vi "HW_QX_Parse Channel Parameters.vi"(8 "error in":errorcluster, 10 "sysModCFG[]":T1[](array[typedef])) -> (0 "error out":errorcluster)   [LabVIEW 2016]
uses:
  Ctrls/HardWare _ Channel Parameters.ctl
  Ctrls/HardWare _ Module Configuration.ctl
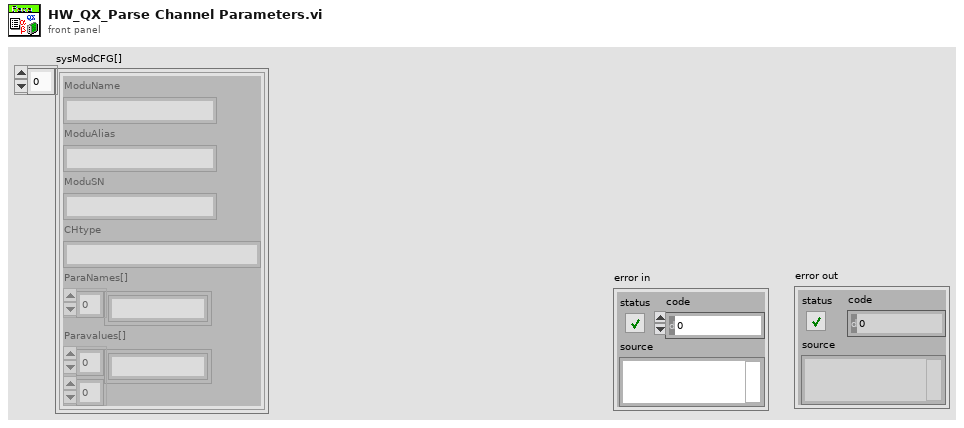
[diagram p1: front panel]
types:
  T1 = typedef "HardWare _ Module Configuration.ctl" = cluster{"ModuName":string, "ModuAlias":string, "ModuSN":string, "CHtype":string, "ParaNames[]":string[], "Paravalues[]":string[][]}
  T2 = typedef "HardWare _ Channel Parameters.ctl" = cluster{"CHType":string[], "CHName":string[], "CHAlias":string[], "Use":bool[], "Unit":string[], "SampleRate":dbl[], "FilterFreq":dbl[], "SlopeA":dbl[], "InterceptB":dbl[], "SampMax":dbl[], "SampMin":dbl[], "AlarmMax":dbl[], "AlarmMin":dbl[]}
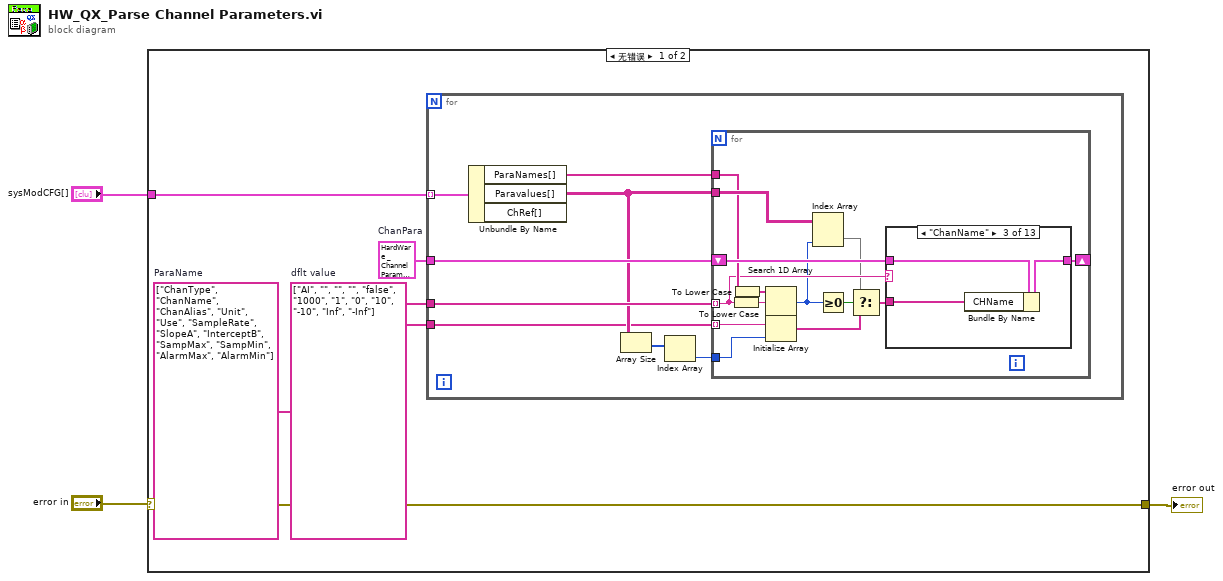
[diagram p0: block diagram]
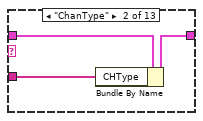
[diagram p3: hidden frame]
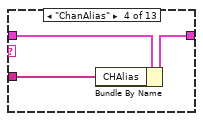
[diagram p4: hidden frame]
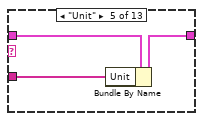
[diagram p5: hidden frame]
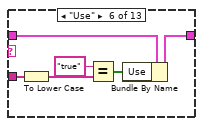
[diagram p6: hidden frame]
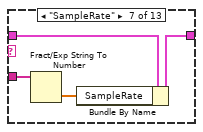
[diagram p7: hidden frame]
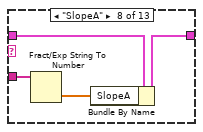
[diagram p8: hidden frame]
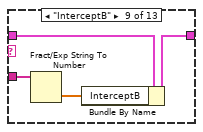
[diagram p9: hidden frame]
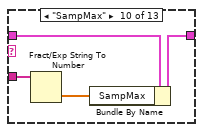
[diagram p10: hidden frame]
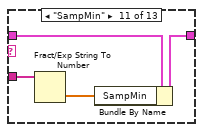
[diagram p11: hidden frame]
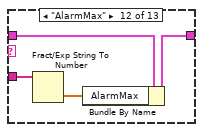
[diagram p12: hidden frame]
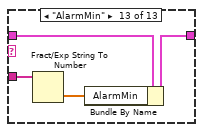
[diagram p13: hidden frame]
diagram:
  n1 = case shown="无错误" "error in" {
    selector: "error in" -> [w4 w78]
    tunnel: "sysModCFG[]" -> [w8 _]
    tunnel: [w4 w78] -> w1
    frame No Error {
      w5 = string[] ["AI", "", "", "", "false", "1000", "1", "0", "10", "-10", "Inf", "-Inf"]  # dflt value
      w6 = string[] ["ChanType", "ChanName", "ChanAlias", "Unit", "Use", "SampleRate", "SlopeA", "InterceptB", "SampMax", "SampMin", "AlarmMax", "AlarmMin"]  # ParaName
      w7 = T2 {"CHType"=[], "CHName"=[], "CHAlias"=[], "Use"=[], "Unit"=[], "SampleRate"=[], "FilterFreq"=[], "SlopeA"=[], "InterceptB"=[], "SampMax"=[], "SampMin"=[], "AlarmMax"=[], "AlarmMin"=[]}  # ChanPara
      n2 = for {
        tunnel: w8 -> [w16] mode=indexing
        tunnel: w7 -> [w14]
        tunnel: w6 -> [w13]
        tunnel: w5 -> [w9]
        n3 = Unbundle By Name(w16) -> ("ParaNames[]"=w15:string[], "Paravalues[]"=w12:string[][])  [unwired: 1 out]
        n4 = Array Size(array=w12) -> (size(s)=w11:i32[])
        n5 = Index Array(array=w11) -> (element=w10:i32)  [unwired: 1 in]
        n6 = for {
          tunnel: w15 -> [w27]
          shift-right: [w28] -> _
          shift-left: w14 -> [w30]
          tunnel: w12 -> [w29]
          tunnel: w13 -> [w26] mode=indexing
          tunnel: w10 -> [w23]
          tunnel: w9 -> [w22] mode=indexing
          n7 = To Lower Case(string=w26) -> (all lower case string=w17:string)
          n8 = To Lower Case(string=w27) -> (all lower case string=w18:string[])
          n9 = Search 1D Array(1D array=w18, element=w17) -> (index of element=w19:i32)  [unwired: 1 in]
          n10 = Initialize Array(w22, w23) -> (w21:string[])
          n11 = Index Array(array=w29, index (col)=w19) -> (element=w24:string[])  [unwired: 1 in]
          n12 = Greater Or Equal To 0?(x=w19) -> (x >= 0?=w25:bool)
          n13 = Select(t=w24, s=w25, f=w21) -> (s? t:f=w20:string[])
          n14 = case shown="\"ChanName\"" w26 {
            tunnel: w30 -> [w31 w34 w37 w40 w43 w49 w53 w57 w61 w65 w69 w73 w77]
            tunnel: w20 -> [_ w32 w36 w39 w42 w48 w51 w55 w59 w63 w67 w71 w75]
            tunnel: [w31 w33 w35 w38 w41 w47 w52 w56 w60 w64 w68 w72 w76] -> w28
            frame Default {
            }
            frame "ChanType" {
              n15 = Bundle By Name(cluster=w34, "CHType"=w32) -> (w33:T2)
            }
            frame "ChanName" {
              n16 = Bundle By Name(cluster=w37, "CHName"=w36) -> (w35:T2)
            }
            frame "ChanAlias" {
              n17 = Bundle By Name(cluster=w40, "CHAlias"=w39) -> (w38:T2)
            }
            frame "Unit" {
              n18 = Bundle By Name(cluster=w43, "Unit"=w42) -> (w41:T2)
            }
            frame "Use" {
              n19 = To Lower Case(string=w48) -> (all lower case string=w46:string[])
              n20 = Equal?(x="true", y=w46) -> (x = y?=w45:bool[])
              n21 = Bundle By Name(cluster=w49, "Use"=w45) -> (w47:T2)
            }
            frame "SampleRate" {
              n22 = Fract/Exp String To Number(string=w51) -> (number=w50:dbl[])  [unwired: 3 in, 1 out]
              n23 = Bundle By Name(cluster=w53, "SampleRate"=w50) -> (w52:T2)
            }
            frame "SlopeA" {
              n24 = Fract/Exp String To Number(string=w55) -> (number=w54:dbl[])  [unwired: 3 in, 1 out]
              n25 = Bundle By Name(cluster=w57, "SlopeA"=w54) -> (w56:T2)
            }
            frame "InterceptB" {
              n26 = Fract/Exp String To Number(string=w59) -> (number=w58:dbl[])  [unwired: 3 in, 1 out]
              n27 = Bundle By Name(cluster=w61, "InterceptB"=w58) -> (w60:T2)
            }
            frame "SampMax" {
              n28 = Fract/Exp String To Number(string=w63) -> (number=w62:dbl[])  [unwired: 3 in, 1 out]
              n29 = Bundle By Name(cluster=w65, "SampMax"=w62) -> (w64:T2)
            }
            frame "SampMin" {
              n30 = Fract/Exp String To Number(string=w67) -> (number=w66:dbl[])  [unwired: 3 in, 1 out]
              n31 = Bundle By Name(cluster=w69, "SampMin"=w66) -> (w68:T2)
            }
            frame "AlarmMax" {
              n32 = Fract/Exp String To Number(string=w71) -> (number=w70:dbl[])  [unwired: 3 in, 1 out]
              n33 = Bundle By Name(cluster=w73, "AlarmMax"=w70) -> (w72:T2)
            }
            frame "AlarmMin" {
              n34 = Fract/Exp String To Number(string=w75) -> (number=w74:dbl[])  [unwired: 3 in, 1 out]
              n35 = Bundle By Name(cluster=w77, "AlarmMin"=w74) -> (w76:T2)
            }
          }
        }
      }
    }
    frame Error {
    }
  }
  "error out" <- w1
